vi "StrQueue-Insert.vi"   [LabVIEW 2015]
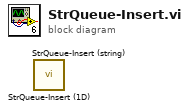
[diagram p0: block diagram]
diagram:
  n1 = call "StrQueue-Insert (1D).vi"() -> ()  [unwired: 5 in, 1 out]
  n2 = call "StrQueue-Insert (string).vi"() -> ()  [unwired: 5 in, 1 out]
